vi "GetDataPackage_Double.vi"(8 "error in (no error)":errorcluster, 11 "VISA Refnum in":refnum<visa-resource-name>) -> (0 "error out":errorcluster, 1 "Raw Data":string, 2 "Data":T1[](array[typedef]), 3 "VISA Refnum out":refnum<visa-resource-name>)   [LabVIEW 2020, in "OXYGEN_Datastream.lvlib"]
uses:
  OXYGEN_Datastream.lvlib
  TypeDefs/DataPoint_Double.ctl
  read_data_package.vi
  parse_package.vi
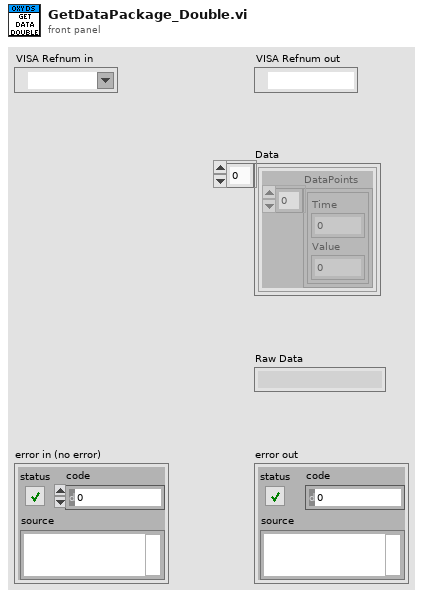
[diagram p1: front panel]
types:
  T1 = typedef "OXYGEN_Datastream.lvlib/DataPoint_Double.ctl" = cluster{"DataPoints":cluster{"Time":dbl, "Value":dbl}[]}
  T2 = typedef "OXYGEN_Datastream.lvlib/DataPoint_Variant.ctl" = cluster{"DataPoints":cluster{"Time":dbl, "Value":variant}[]}
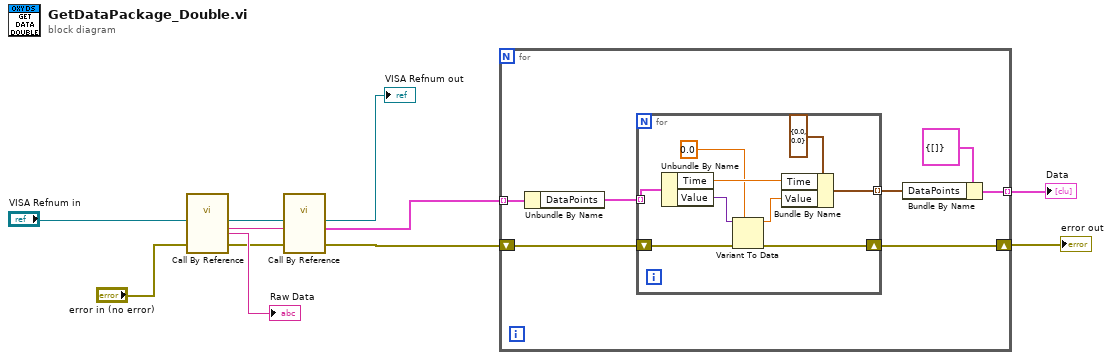
[diagram p0: block diagram]
diagram:
  n1 = call-by-ref "?"("error in (no error)"="error in (no error)", "OXY_SCPI Reseource In"="VISA Refnum in") -> ("error out"=w1:errorcluster, "Complete Raw data"=→"Raw Data":string, "Package without Header"=w8:string, "OXY_SCPI Reseource Out"=w7:refnum<visa-resource-name>)  [unwired: 8 in, 2 out]
  n2 = call-by-ref "?"("error in (no error)"=w1, "Raw Package without Header"=w8, "OXY_SCPI Reseource In"=w7) -> ("error out"=w5:errorcluster, "DataAllChannels"=w6:T2[], "OXY_SCPI Reseource Out"=→"VISA Refnum out":refnum<visa-resource-name>)  [unwired: 8 in, 2 out]
  n3 = for {
    tunnel: w6 -> [w18] mode=indexing
    shift-right: [w15] -> w4
    shift-left: w5 -> [w16]
    tunnel: [w12] -> w3 mode=indexing
    n4 = Unbundle By Name(w18) -> ("DataPoints"=w17:cluster{"Time":dbl, "Value":variant}[])
    n5 = for {
      tunnel: w17 -> [w27] mode=indexing
      shift-right: [w23] -> w15
      shift-left: w16 -> [w24]
      tunnel: [w22] -> w13 mode=indexing
      n6 = Unbundle By Name(w27) -> ("Time"=w25:dbl, "Value"=w21:variant)
      n7 = Variant To Data(error in=w24, type=0.0, Variant=w21) -> (data=w19:dbl, error out=w23:errorcluster)
      n8 = Bundle By Name(cluster=cluster{"Time":dbl, "Value":dbl} {"Time"=0.0, "Value"=0.0}, "Time"=w25, "Value"=w19) -> (w22:cluster{"Time":dbl, "Value":dbl})
    }
    n9 = Bundle By Name(cluster=T1 {"DataPoints"=[]} ("Data"), "DataPoints"=w13) -> (w12:T1)
  }
  "error out" <- w4
  "Data" <- w3
